vi "GET POV DEFAULTS.vi"(11 "Cluster":T5={"RefAngle"="", "RefSetAngle"="", "ServoDeviceRef"={"DeviceStatus"={"status"=FALSE, "code"=0, "source"=""}, "PWM Channel"=enum."Invalid", "DeadBand"={"Name"="", "maxPositivePwm"=0, "minPositivePwm"=0, "centerPwm"=0, "maxNegativePwm"=0, "minNegativePwm"=0, "angularRange"=0}}}) -> (3 "Array":T4(array[cluster]))   [LabVIEW 2020]
uses:
  <vilib>/Rock Robotics/WPI/PWM/Servo/WPI_ServoDeviceRef.ctl
  <vilib>/Rock Robotics/SystemInterfaces/DIO/FPGA_DIOPWMChannel.ctl
  <vilib>/Rock Robotics/WPI/PWM/WPI_PWMDeadband.ctl
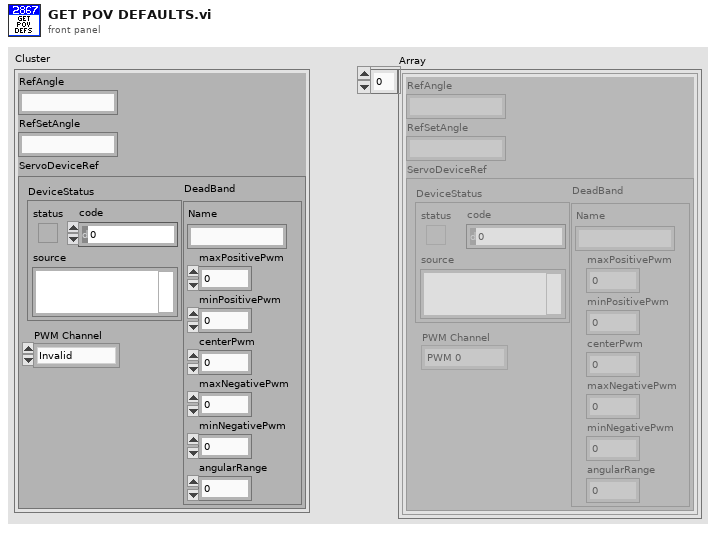
[diagram p1: front panel]
types:
  T1 = typedef "WPI_ServoDeviceRef.ctl" = cluster{"DeviceStatus":errorcluster, "PWM Channel":T2, "DeadBand":T3}
  T2 = typedef "FPGA_DIOPWMChannel.ctl" = enum8{"PWM 0", "PWM 1", "PWM 2", "PWM 3", "PWM 4", "PWM 5", "PWM 6", "PWM 7", "PWM 8", "PWM 9", "PWM MXP 0", "PWM MXP 1", "PWM MXP 2", "PWM MXP 3", "PWM MXP 4", "PWM MXP 5", "PWM MXP 6", "PWM MXP 7", "PWM MXP 8", "PWM MXP 9", "Invalid"}
  T3 = typedef "WPI_PWMDeadband.ctl" = cluster{"Name":string, "maxPositivePwm":i32, "minPositivePwm":i32, "centerPwm":i32, "maxNegativePwm":i32, "minNegativePwm":i32, "angularRange":u16}
  T4 = cluster{"RefAngle":string, "RefSetAngle":string, "ServoDeviceRef":T1}[]
  T5 = cluster{"RefAngle":string, "RefSetAngle":string, "ServoDeviceRef":T1}
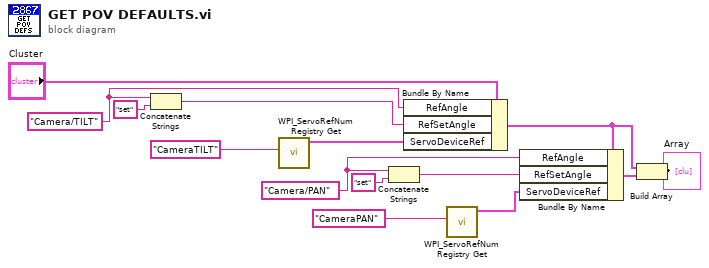
[diagram p0: block diagram]
diagram:
  w11 = "Camera/PAN" ("Name")
  w6 = "Camera/TILT" ("Name")
  n1 = Concatenate Strings(w6, "set" ("string")) -> (w5:string)
  n2 = call <vilib>:"WPI_ServoRefNum Registry Get.vi"("refnum name"="CameraTILT") -> ("ServoDeviceRef"=w9:T1)  [unwired: 9 in, 1 out]
  n3 = Concatenate Strings(w11, "set" ("string")) -> (w10:string)
  n4 = Bundle By Name(cluster="Cluster", "RefAngle"=w6, "RefSetAngle"=w5, "ServoDeviceRef"=w9) -> (w3:T5)
  n5 = call <vilib>:"WPI_ServoRefNum Registry Get.vi"("refnum name"="CameraPAN") -> ("ServoDeviceRef"=w14:T1)  [unwired: 9 in, 1 out]
  n6 = Bundle By Name(cluster=w3, "RefAngle"=w11, "RefSetAngle"=w10, "ServoDeviceRef"=w14) -> (w2:T5)
  n7 = Build Array(w3, w2) -> (→"Array":T4)
